vi "String to Modbus.vi"(10 "String":string) -> (1 "Array":u16[](array[numeric]))   [LabVIEW 2024, in "Bronkhorst Flexi-Flow ModbusTCP API.lvlib"]
uses:
  Bronkhorst Flexi-Flow ModbusTCP API.lvlib
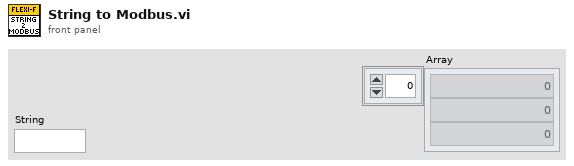
[diagram p1: front panel]
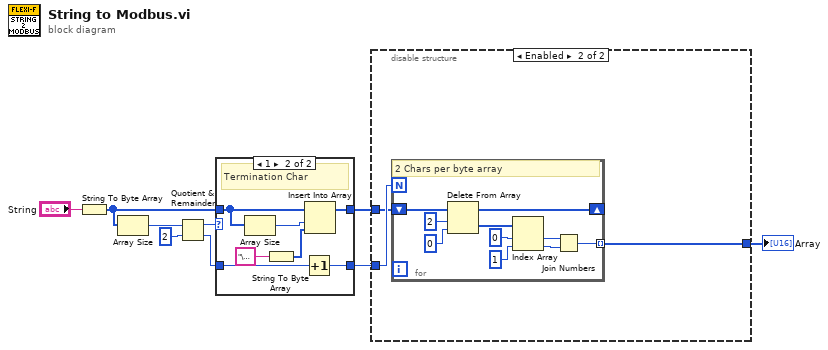
[diagram p0: block diagram]
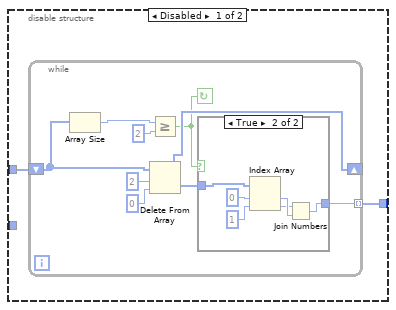
[diagram p3: hidden frame]
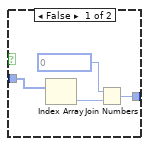
[diagram p4: hidden frame]
diagram:
  n1 = String To Byte Array(string="String") -> (unsigned byte array=w3:u8[])
  n2 = Array Size(array=w3) -> (size(s)=w7:i32)
  n3 = Quotient & Remainder(x=w7, y=2) -> (x-y*floor(x/y)=w5:i32, floor(x/y)=w2:i32)
  n4 = case shown="1" w5 {
    tunnel: [w11 w16] -> w4
    tunnel: w3 -> [w11 w18]
    tunnel: w2 -> [w10 w15]
    tunnel: [w10 w14] -> w1
    frame 0, Default {
    }
    frame 1 {
      # "Termination Char"
      n5 = Array Size(array=w18) -> (size(s)=w17:i32)
      n6 = String To Byte Array(string="\u0000") -> (unsigned byte array=w12:u8[])
      n7 = Increment(x=w15) -> (x+1=w14:i32)
      n8 = Insert Into Array(array=w18, index=w17, new element=w12) -> (w16:u8[])
    }
  }
  n9 = disable-structure shown="Enabled" {
    disable-tunnel: w4 -> [w20 w41]
    disable-tunnel: [w19 w40] -> w8
    disable-tunnel: w1 -> [_ w42]
    frame Disabled {
      n10 = while {
        tunnel: [w23] -> w19 mode=indexing
        shift-right: [w28] -> _
        shift-left: w20 -> [w27]
        stop <- w22 continue-if-true
        n11 = Array Size(array=w27) -> (size(s)=w26:i32)
        n12 = Greater Or Equal?(x=w26, y=2 ("length")) -> (x >= y?=w22:bool)
        n13 = Delete From Array(array=w27, length=2, index=0) -> (deleted portion=w24:u8[], array with subset deleted=w28:u8[])
        n14 = case shown="True" w22 {
          tunnel: w24 -> [w31 w39]
          tunnel: [w32 w34] -> w23
          frame False {
            n15 = Index Array(array=w31) -> (element=w30:u8)  [unwired: 1 in]
            n16 = Join Numbers(hi=u8 0, lo=w30) -> ((hi.lo)=w32:u16)
          }
          frame True {
            n17 = Index Array(array=w39, index #1=0 ("index"), index #2=1 ("index")) -> (element #1=w36:u8, element #2=w35:u8)
            n18 = Join Numbers(hi=w35, lo=w36) -> ((hi.lo)=w34:u16)
          }
        }
      }
    }
    frame Enabled {
      n19 = for {
        N: w42 -> [_]
        tunnel: [w49] -> w40 mode=indexing
        shift-right: [w46] -> _
        shift-left: w41 -> [w48]
        # "2 Chars per byte array"
        n20 = Delete From Array(array=w48, length=2, index=0) -> (deleted portion=w47:u8[], array with subset deleted=w46:u8[])
        n21 = Index Array(array=w47, index #1=0 ("index"), index #2=1 ("index")) -> (element #1=w45:u8, element #2=w44:u8)
        n22 = Join Numbers(hi=w45, lo=w44) -> ((hi.lo)=w49:u16)
      }
    }
  }
  "Array" <- w8
